vi "Auto Shoot.vi"(0 "Finished Crossing":bool, 1 "Linear Velocity":dbl=0.4 format="%#_13g", 3 "Rotational Velocity":dbl=0.1 format="%#_13g", 5 "Edge Detected":bool, 9 "Ball In":bool, 12 "Max Coordinate":i32[](array[numeric]), 13 "Image Size":i32[](array[numeric])) -> (4 "Translational Velocity Deployed":dbl, 6 "Rotational Velocity Deployed":dbl, 8 "Done":bool=TRUE, 10 "Shooter":dbl, 15 "Intake":dbl)   [LabVIEW 2015]
uses:
  Auto Shooting with Vision.ctl
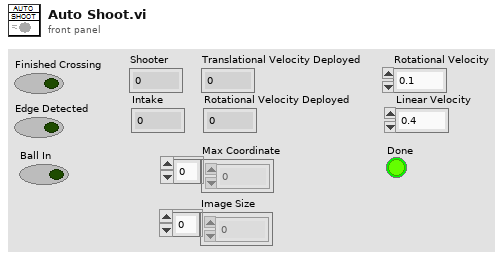
[diagram p1: front panel]
types:
  T1 = typedef "Auto Shooting with Vision.ctl" = enum16{"Ready", "Move Forward", "Vision Tracking", "Shoot", "Done"}
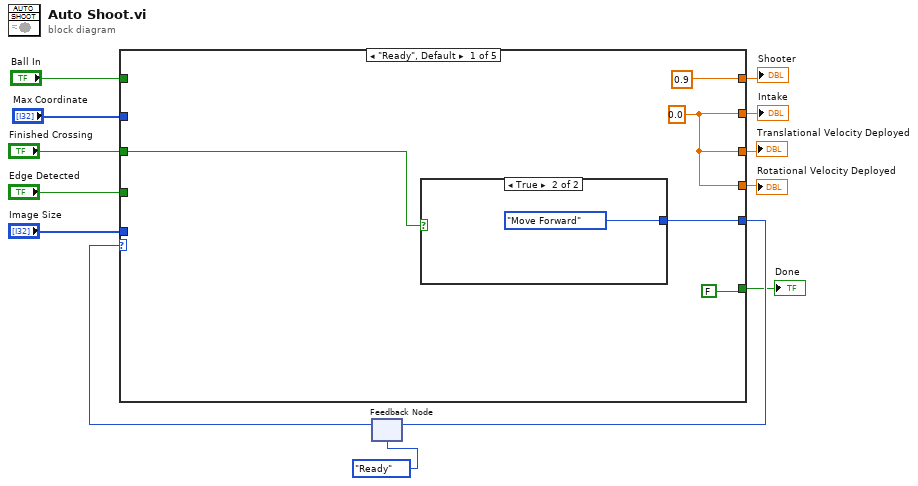
[diagram p0: block diagram]
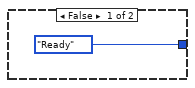
[diagram p2: hidden frame]
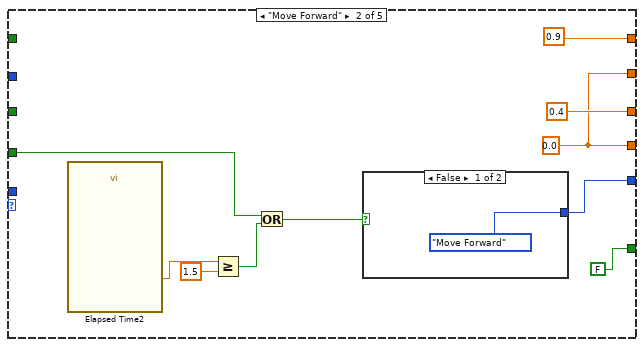
[diagram p3: hidden frame]
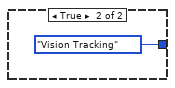
[diagram p4: hidden frame]
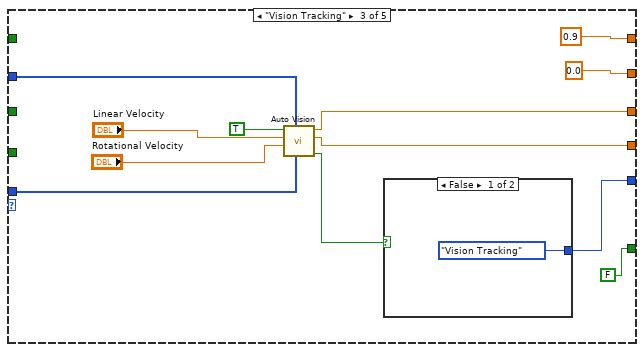
[diagram p5: hidden frame]
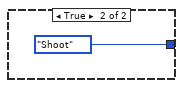
[diagram p6: hidden frame]
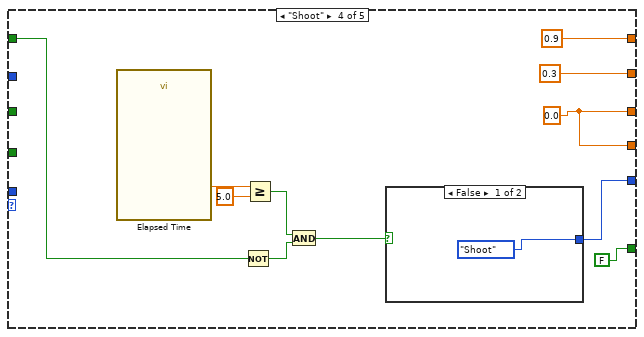
[diagram p7: hidden frame]
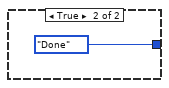
[diagram p8: hidden frame]
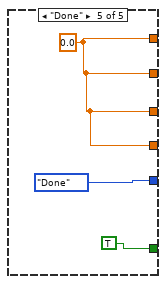
[diagram p9: hidden frame]
diagram:
  n1 = feedback #1(Auto_Shooting_with_Vision."Ready") -> (w12:T1)
  n2 = case shown="\"Ready\", Default" w12 {
    tunnel: "Finished Crossing" -> [w18 _ _ _ _]
    tunnel: [w17 w30 w37 w56 Auto_Shooting_with_Vision."Done"] -> w10
    tunnel: "Edge Detected" -> [_ w25 _ _ _]
    tunnel: [w16 0.4 w41 w57 w61] -> w8
    tunnel: [w16 w27 w40 w57 w61] -> w7
    tunnel: "Max Coordinate" -> [_ _ w39 _ _]
    tunnel: "Image Size" -> [_ _ w38 _ _]
    tunnel: "Ball In" -> [_ _ _ w55 _]
    tunnel: [0.9 0.9 0.9 0.9 w61] -> w3
    tunnel: [w16 w27 0.0 0.3 w61] -> w2
    tunnel: [FALSE FALSE FALSE FALSE TRUE] -> w1
    frame "Ready", Default {
      w16 = 0.0
      n3 = case shown="True" w18 {
        tunnel: [Auto_Shooting_with_Vision."Ready" Auto_Shooting_with_Vision."Move Forward"] -> w17
        frame False {
        }
        frame True {
        }
      }
    }
    frame "Move Forward" {
      w27 = 0.0
      n4 = call "Elapsed Time2"() -> ("Elapsed Time (s)"=w23:dbl)  [unwired: 12 in, 7 out]
      n5 = Greater Or Equal?(x=w23, y=1.5) -> (x >= y?=w21:bool)
      n6 = Or(x=w25, y=w21) -> (x .or. y?=w24:bool)
      n7 = case shown="False" w24 {
        tunnel: [Auto_Shooting_with_Vision."Move Forward" Auto_Shooting_with_Vision."Vision Tracking"] -> w30
        frame False {
        }
        frame True {
        }
      }
    }
    frame "Vision Tracking" {
      n8 = call "Auto Vision.vi"("Image Size"=w38, "Max Coordinate"=w39, "Rotational Velocity"="Rotational Velocity", "Linear Velocity"="Linear Velocity", "Follow Colour ON"=TRUE) -> ("Done"=w33:bool, "Rotational Velocity_After"=w40:dbl, "Translational Velocity_After"=w41:dbl)  [unwired: 4 in]
      n9 = case shown="False" w33 {
        tunnel: [Auto_Shooting_with_Vision."Vision Tracking" Auto_Shooting_with_Vision."Shoot"] -> w37
        frame False {
        }
        frame True {
        }
      }
    }
    frame "Shoot" {
      w57 = 0.0
      n10 = call "Elapsed Time"() -> ("Elapsed Time (s)"=w53:dbl)  [unwired: 12 in, 7 out]
      n11 = Not(x=w55) -> (.not. x?=w54:bool)
      n12 = Greater Or Equal?(x=w53, y=5.0) -> (x >= y?=w51:bool)
      n13 = And(x=w51, y=w54) -> (x .and. y?=w50:bool)
      n14 = case shown="False" w50 {
        tunnel: [Auto_Shooting_with_Vision."Shoot" Auto_Shooting_with_Vision."Done"] -> w56
        frame False {
        }
        frame True {
        }
      }
    }
    frame "Done" {
      w61 = 0.0
    }
  }
  "Translational Velocity Deployed" <- w8
  "Rotational Velocity Deployed" <- w7
  "Shooter" <- w3
  "Intake" <- w2
  "Done" <- w1
  n15 = feedback-in #1(w10) -> ()
